vi "Close Device.vi"(8 "error in (no error)":errorcluster, 11 "CS++DeviceActor in":refnum<class "CS++DeviceActor.lvclass">) -> (0 "error out":errorcluster, 3 "CS++DeviceActor out":refnum<class "CS++DeviceActor.lvclass">)   [LabVIEW 2015, in "CS++DeviceActor.lvlib" / "CS++DeviceActor.lvclass"]
doc: "Close device driver connection."
uses:
  CS++DeviceActor.lvclass
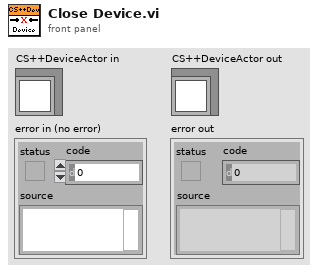
[diagram p1: front panel]
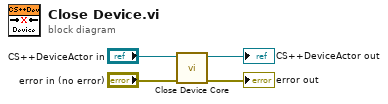
[diagram p0: block diagram]
diagram:
  n1 = call-dynamic "Close Device Core.vi"("error in (no error)"="error in (no error)", "CS++DeviceActor in"="CS++DeviceActor in") -> ("error out"=→"error out":errorcluster, "CS++DeviceActor out"=→"CS++DeviceActor out":refnum<class "CS++DeviceActor.lvclass">)  [unwired: 8 in]
